vi "Method.vi"(4 "Value":refnum<class "Abs_I64 Integer.lvclass">) -> (1 "Result":refnum<class "Abs_I64 Integer.lvclass">)   [LabVIEW 2021, in "Increment_I64.lvclass"]
uses:
  Increment_I64.lvclass
  Abs_Types/I64 Integer/Abs_I64 Integer.lvclass
  C:/Users/Tim/Documents/LabVIEW/2021/Data Classes/Source/Functions/Support/One Terminal/I64/AbsFunc_One Term_I64.lvclass
  C:/Users/Tim/Documents/LabVIEW/2021/Data Classes/Source/Abs_Types/I64 Integer/Abs_I64 Integer.lvclass
  Support/One Terminal/I64/AbsFunc_One Term_I64.lvclass/AbsFunc_One Term_I64.ctl
  Support/One Terminal/I64/Properties/Write Numeric A.vi
  Increment_I64.lvclass/Increment_I64.ctl
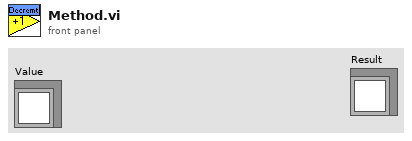
[diagram p1: front panel]
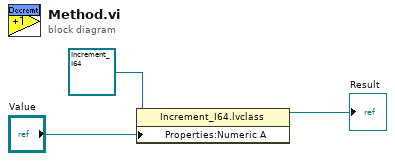
[diagram p0: block diagram]
diagram:
  n1 = property class="Increment_I64.lvclass"(reference=refnum<class "Increment_I64.lvclass"> refnum ("Decrement_DBL.lvclass"), "Properties:Numeric A"="Value") -> (reference out=→"Result":refnum<class "Increment_I64.lvclass">)  [unwired: 1 in, 1 out]
